vi "Module_UI_SnakeClient.vi"(8 "error in (no error)":errorcluster, 10 "Wait on Module(s) (\"\": none)":string) -> (0 "error out":errorcluster)   [LabVIEW 2019, in "Module_UI_SnakeClient.lvclass"]
doc: "created using\nJSMA Module Template - UI Class 0.3.0.13\nRob Humfeld - Jet Engineering\nCopyright (c) 2020, Jet Engineering"
uses:
  Module_UI_SnakeClient.lvclass
  Private/Module_UI_SnakeClient_jMsgRxList STYP.ctl
  <userlib>/JET Engineering/JSMA Standard Messages/jMsg_Sys_UIPanelOpen/jMsg_Sys_UIPanel_Open.lvclass
  C:/Program Files/National Instruments/LabVIEW 2019/user.lib/Jet Engineering/JSMA/Libraries/jMsg Class/jMsg.lvclass
  Private/Module_UI_SnakeClient_jMsgTxList STYP.ctl
  <userlib>/Jet Engineering/JSMA/Libraries/jMsg_CORE/jMsg_JSMA_ApplicationShutdown/jMsg_JSMA_ApplicationShutdown.lvclass
  C:/Program Files/National Instruments/LabVIEW 2019/user.lib/Jet Engineering/JSMA/Libraries/jModule Class/jModule.lvclass
  Private/Module_UI_SnakeClient_LocalData STYP.ctl
  <userlib>/Jet Engineering/JSMA/Libraries/jModule Class/jModule.lvclass/jModule.ctl
  Module_UI_SnakeClient.lvclass/Module_UI_SnakeClient.ctl
  <userlib>/JET Engineering/JSMA Standard Messages/jMsg_Sys_UIPanelOpen/jMsg_Sys_UIPanel_Open.lvclass/jMsg_Sys_UIPanel_Open.ctl
  <userlib>/Jet Engineering/JET_QSM/Code/Private/JET_QSM - Add State [String API].vi
  <userlib>/Jet Engineering/JET_QSM/Code/Private/JET_QSM - Add State to Front [String API].vi
  <userlib>/Jet Engineering/JSMA/Libraries/jModule Class/jModule - Set Static Timer.vi
  <userlib>/Jet Engineering/JSMA/Libraries/jModule Class/jModule - Set Periodic Timer.vi
  <userlib>/Jet Engineering/JSMA/Libraries/jModule Class/Read jMsgRx.vi
  <vilib>/Utility/error.llb/Trim Whitespace.vi
  <vilib>/Utility/error.llb/Error Cluster From Error Code.vi
  <userlib>/Jet Labs/JET Panel/JETPanel.lvclass
  <userlib>/Jet Engineering/JSMA/Libraries/jModule Class/jModule.lvclass
panel:
  out "winSizer B":string="W"
  out "winSizer A":string="W"
  out "jModule Name":string
  out "Recent states before Error (with tick counts) 2":string="0.167 sec ago: VI Initialize\n0.167 sec ago: Window Open\n0.110 sec ago: Control Update\n0.110 sec ago: Indicator Update\n0.000 sec ago: Error Handler\r\n"
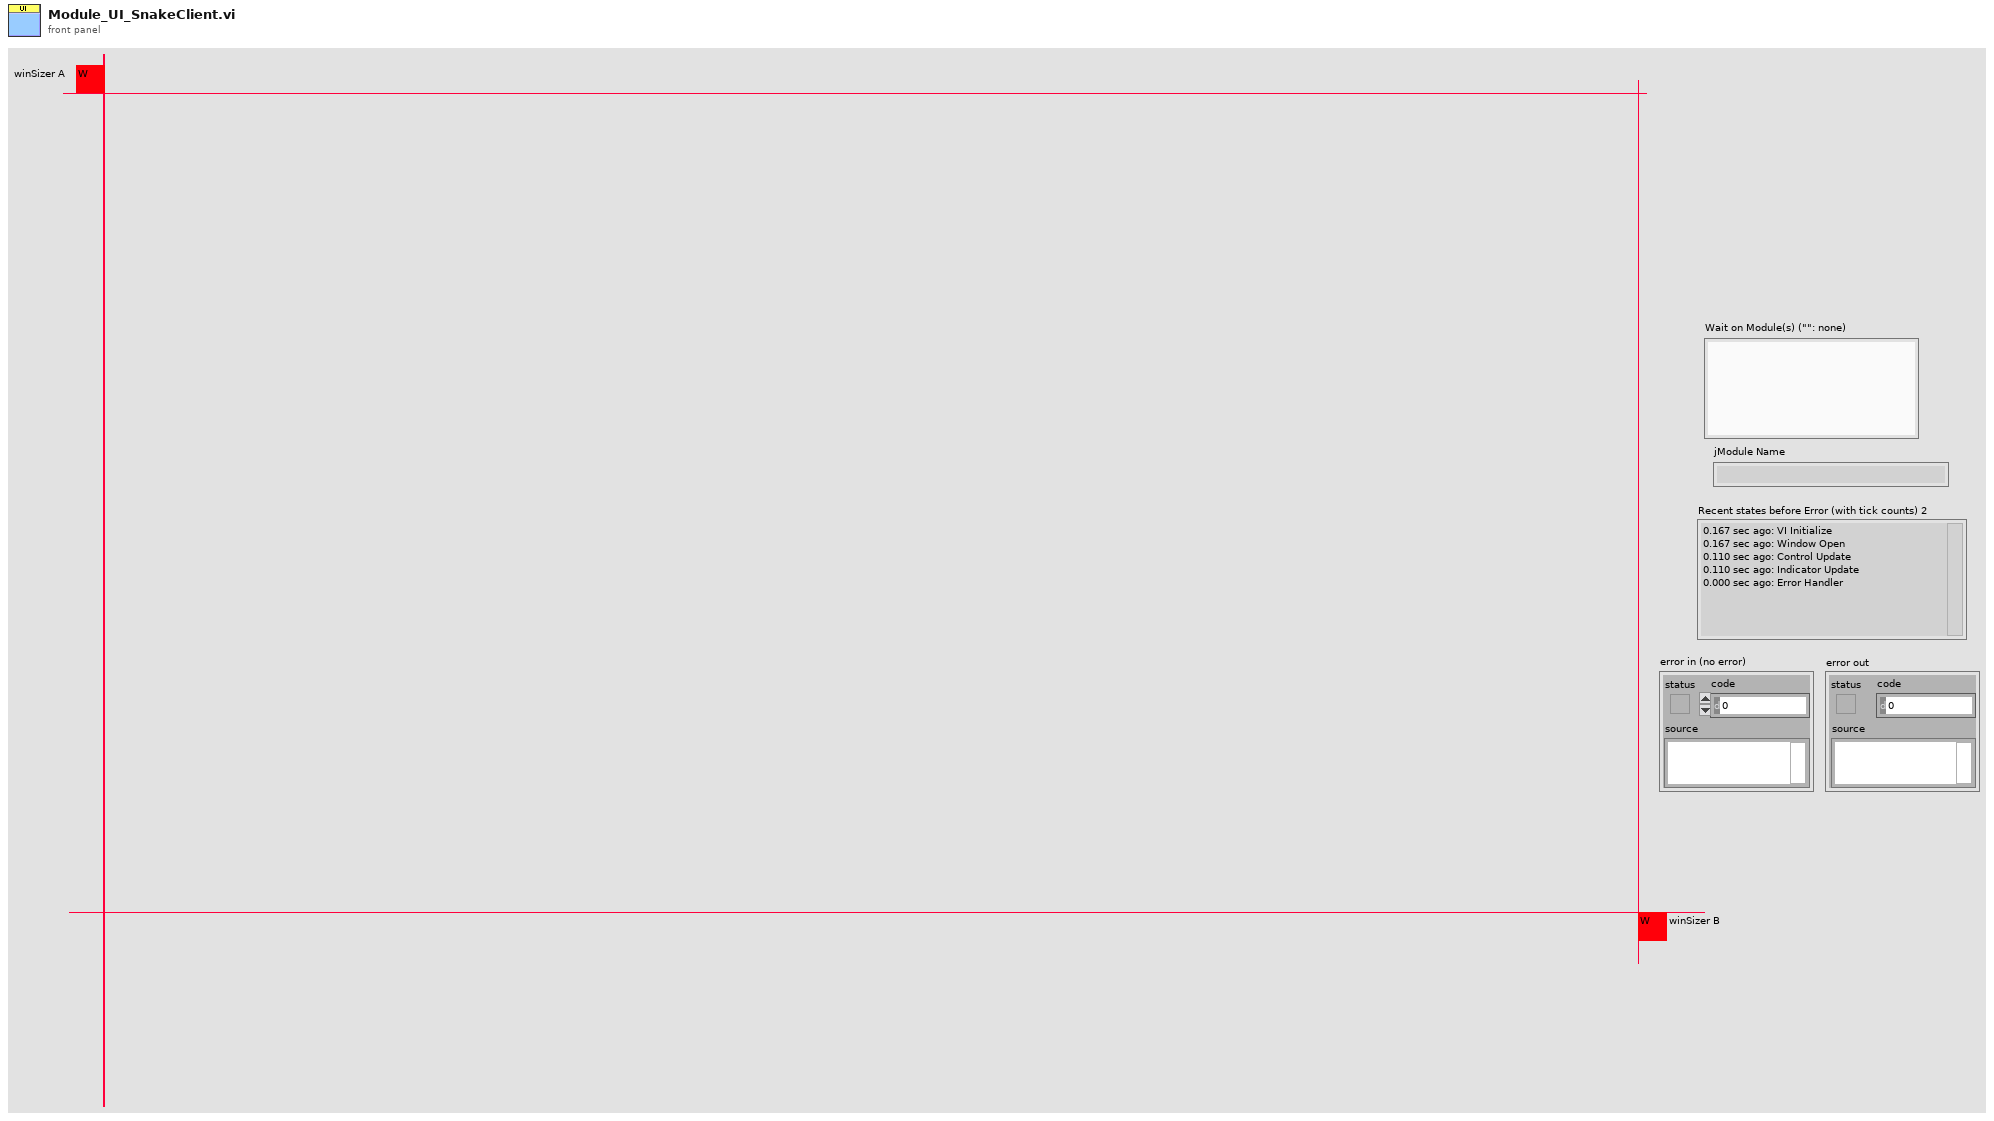
[diagram p1: front panel]
types:
  T1 = typedef "Module_UI_SnakeClient.lvclass/Module_UI_SnakeClient_LocalData STYP.ctl" = cluster{"VI":cluster{"error":errorcluster, "isExiting?":bool}, "UI":cluster{"<placeholder>":bool}}
  T2 = typedef "Module_UI_SnakeClient.lvclass/Module_UI_SnakeClient_jMsgTxList STYP.ctl" = cluster{"jMsg_JSMA_ApplicationShutdown":refnum<class "jMsg_JSMA_ApplicationShutdown.lvclass">}
  T3 = typedef "Module_UI_SnakeClient.lvclass/Module_UI_SnakeClient_jMsgRxList STYP.ctl" = cluster{"jMsg_Sys_UIPanel_Open":refnum<class "jMsg_Sys_UIPanel_Open.lvclass">}
  T4 = typedef "JET_QSM_Refnum STYP.ctl" = cluster{"state":cluster{"queue":refnum<queue>, "idle":string, "error":string, "STOP":string}, "debug":cluster{"enabled?":bool, "queue":refnum<queue>}, "Invalid.option":T5, "QSM.Name":string}
  T5 = typedef "JET_QSM_InvalidOption STYP.ctl" = enum16{"Ignore", "Dialog", "Error"}
  T6 = typedef "JET_QSM_Element STYP.ctl" = cluster{"state":string, "data":variant, "comment":string}
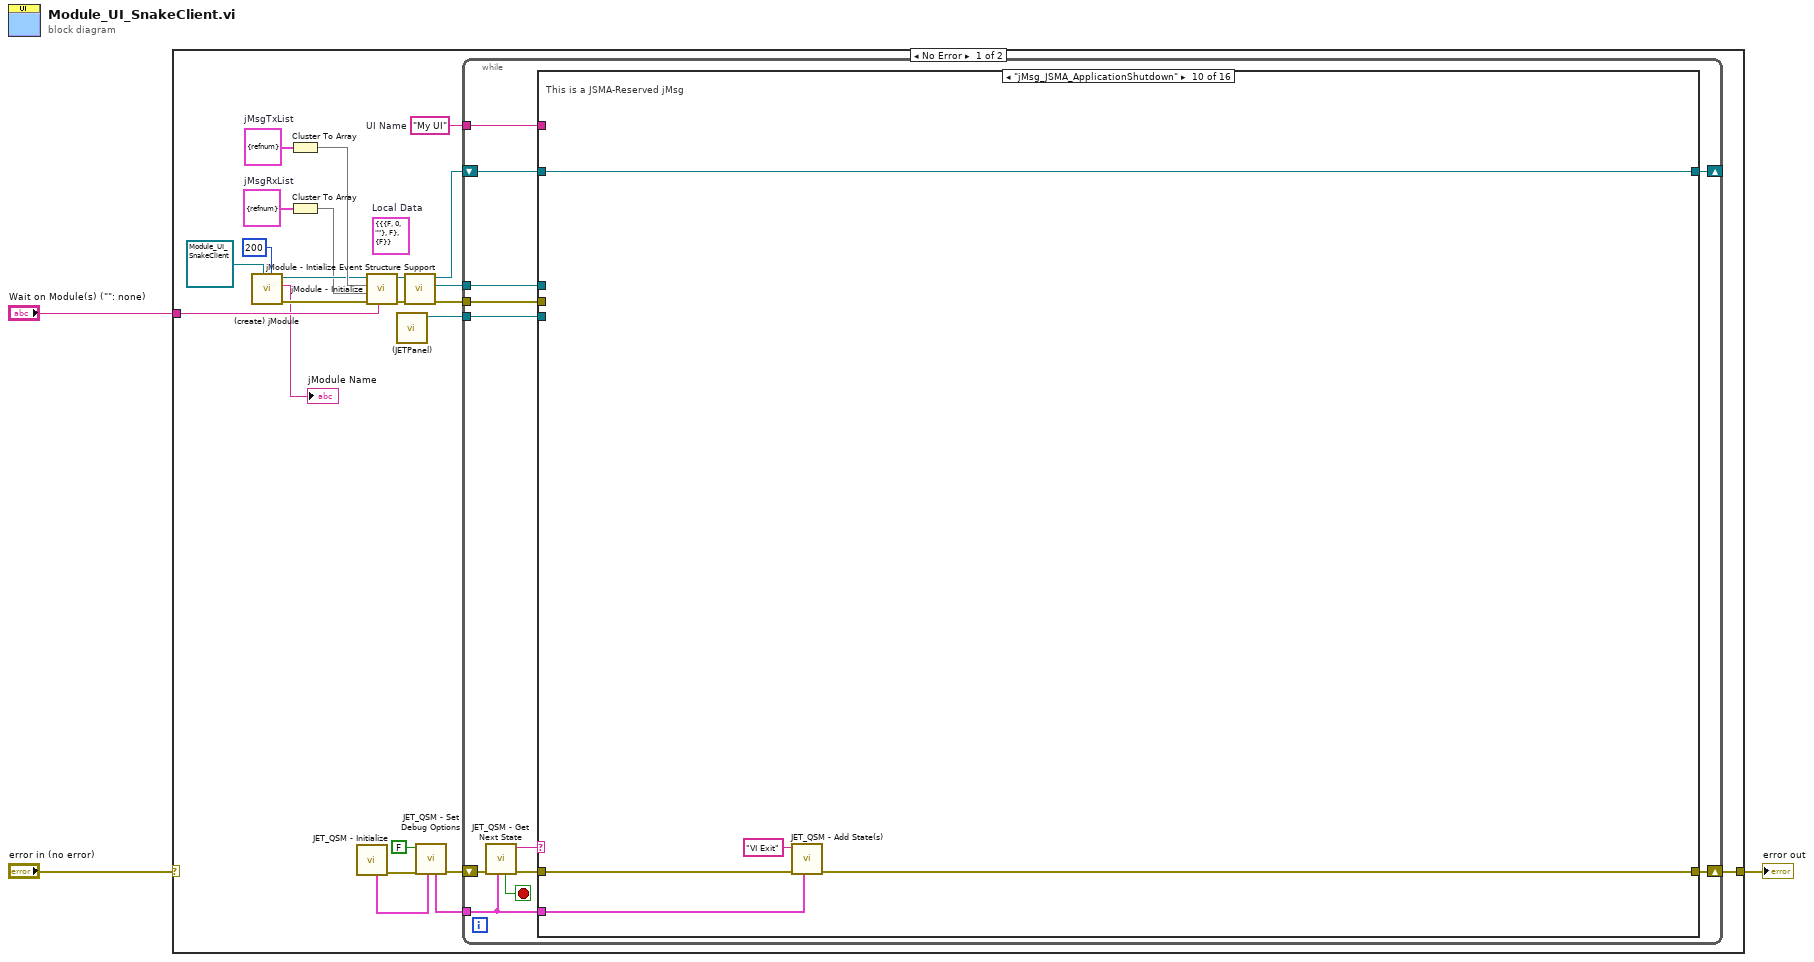
[diagram p0: block diagram]
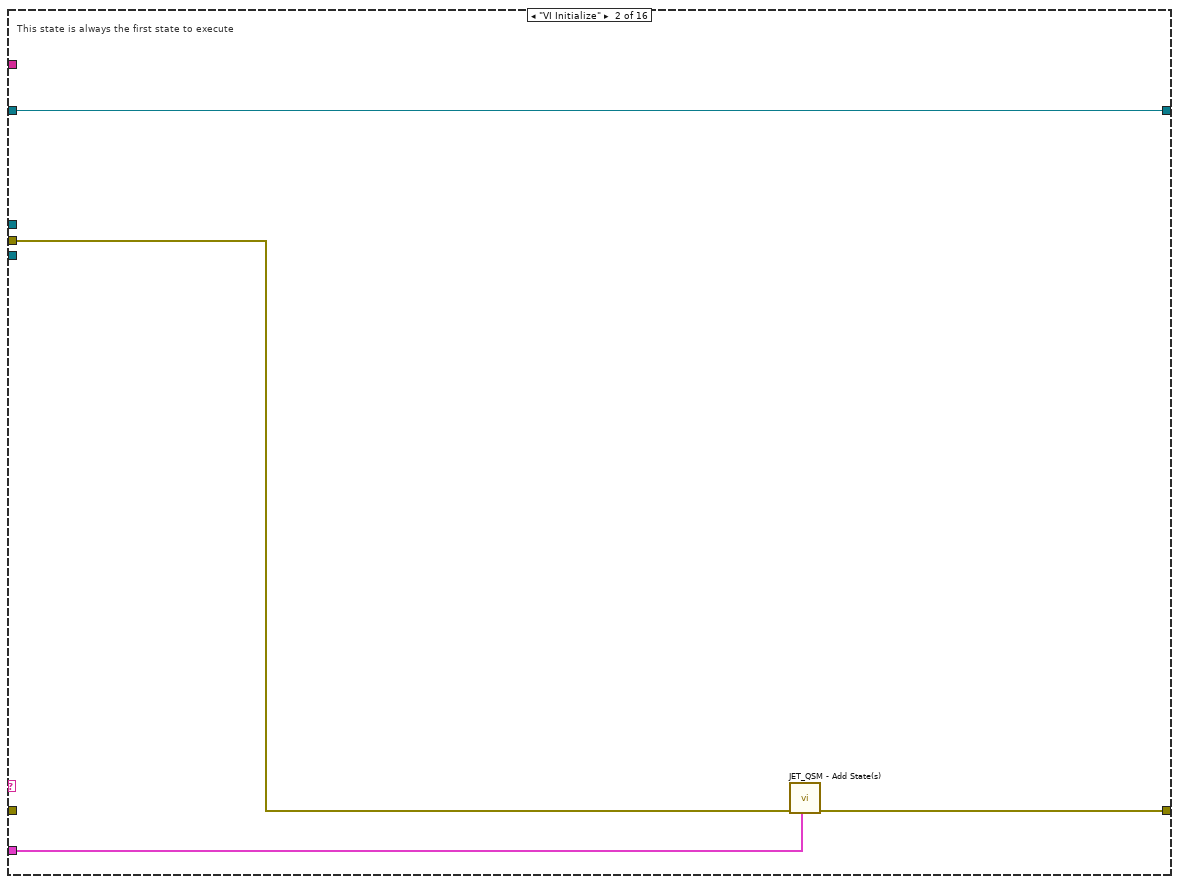
[diagram p3: hidden frame]
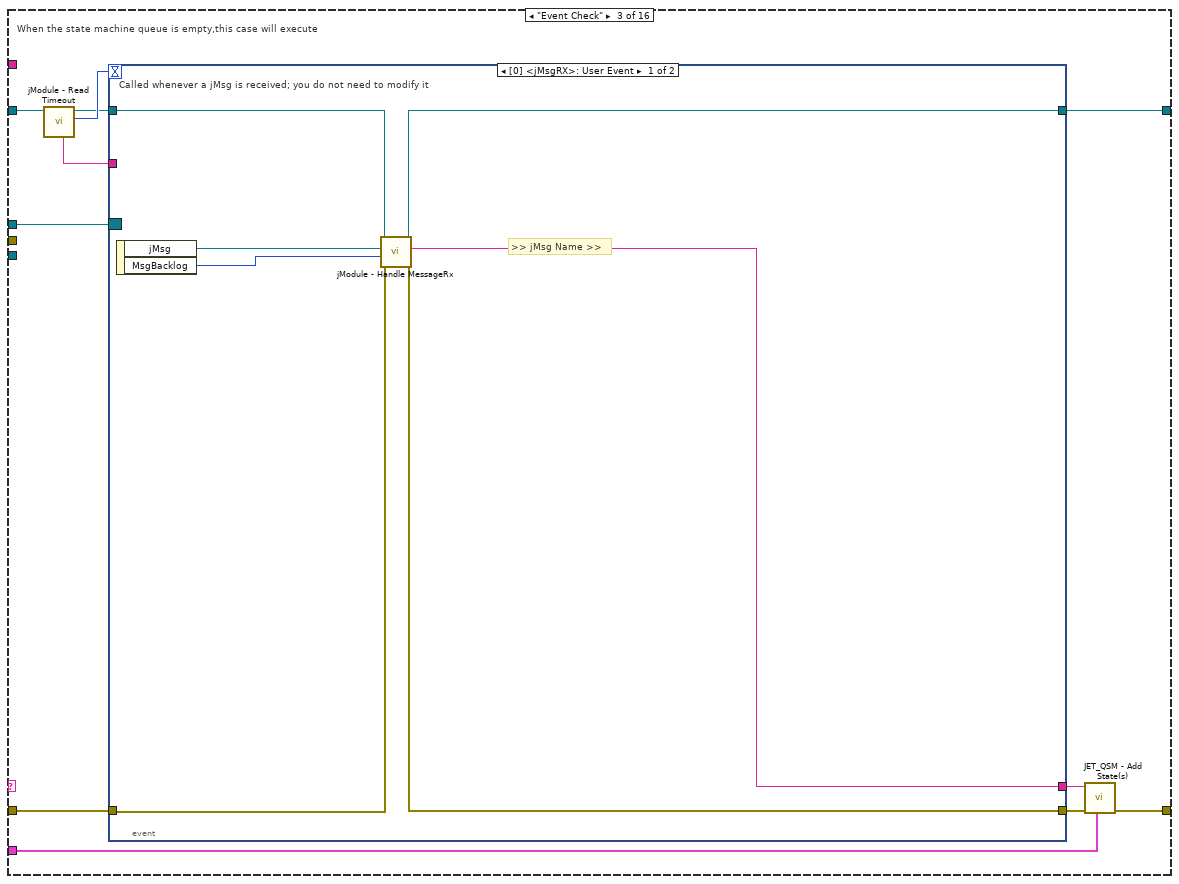
[diagram p4: hidden frame]
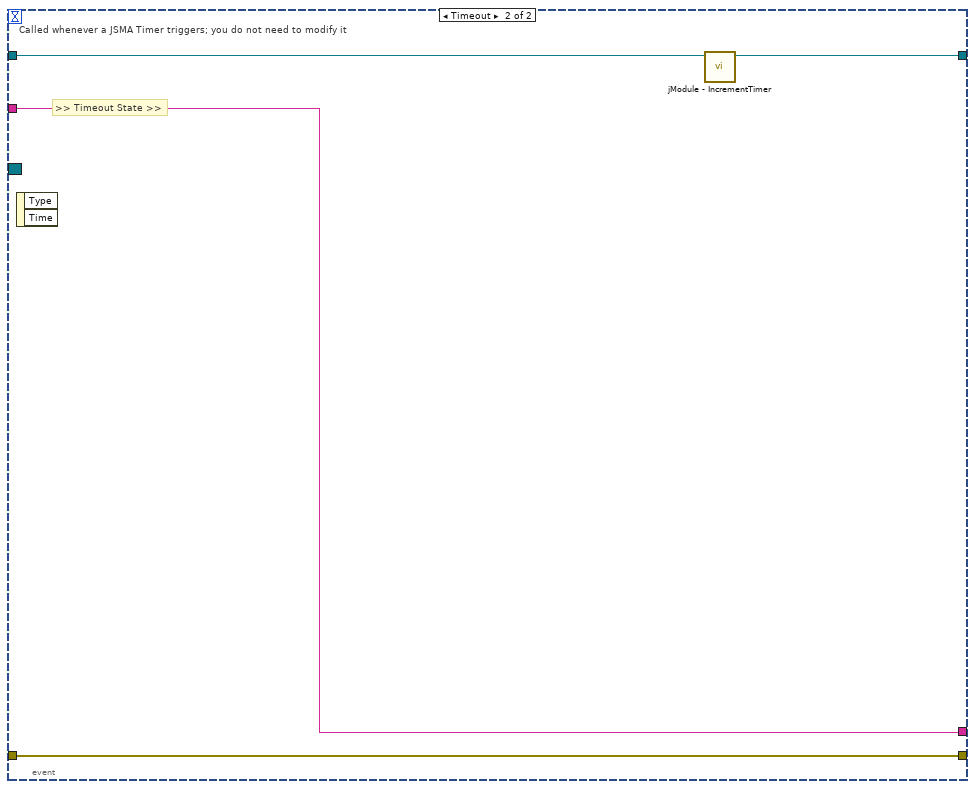
[diagram p5: hidden frame]
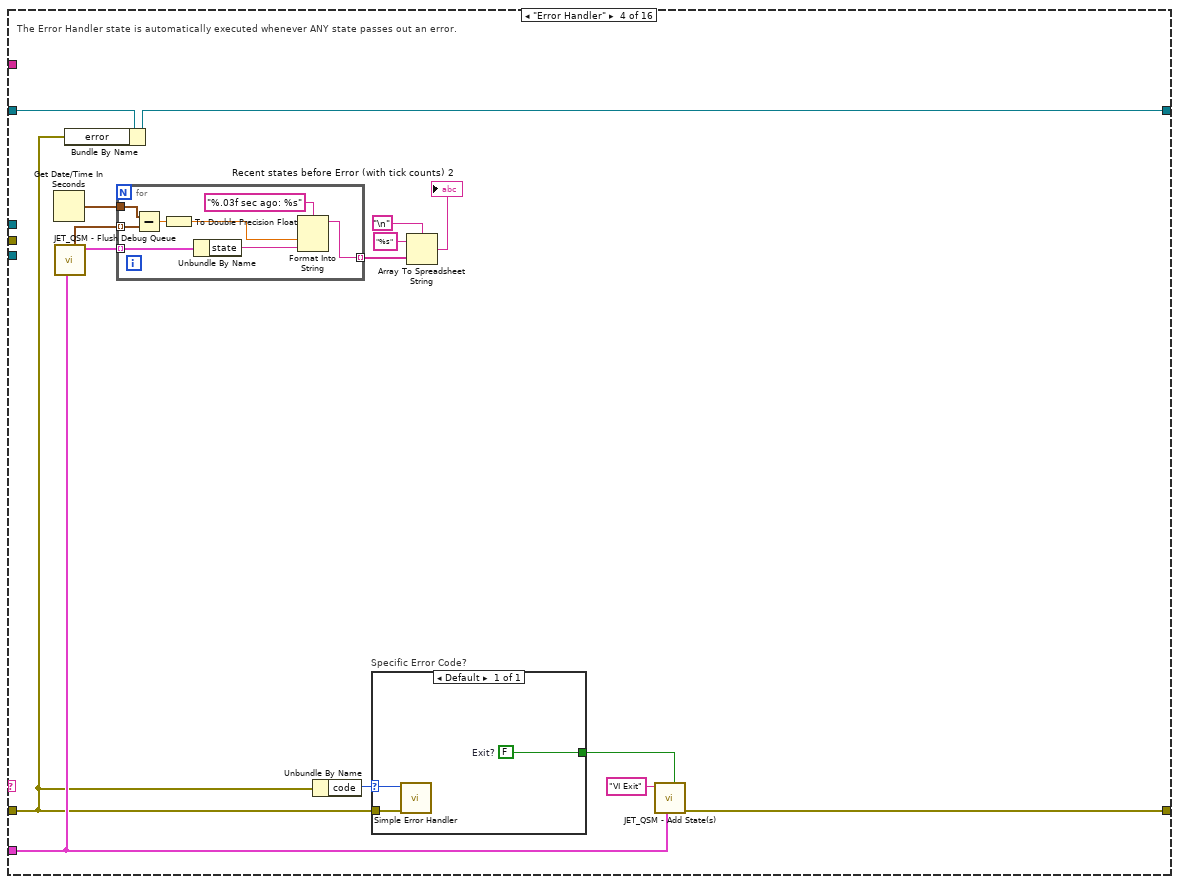
[diagram p6: hidden frame]
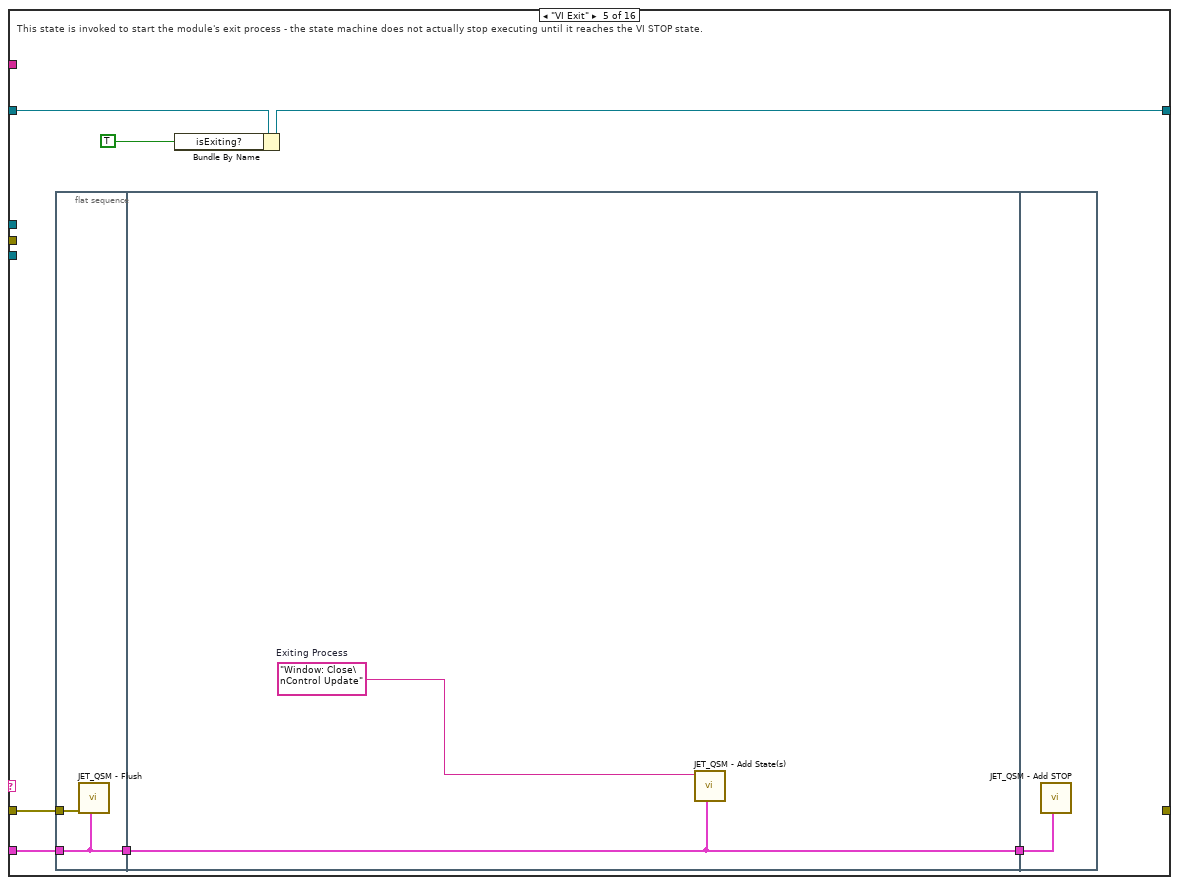
[diagram p7: hidden frame]
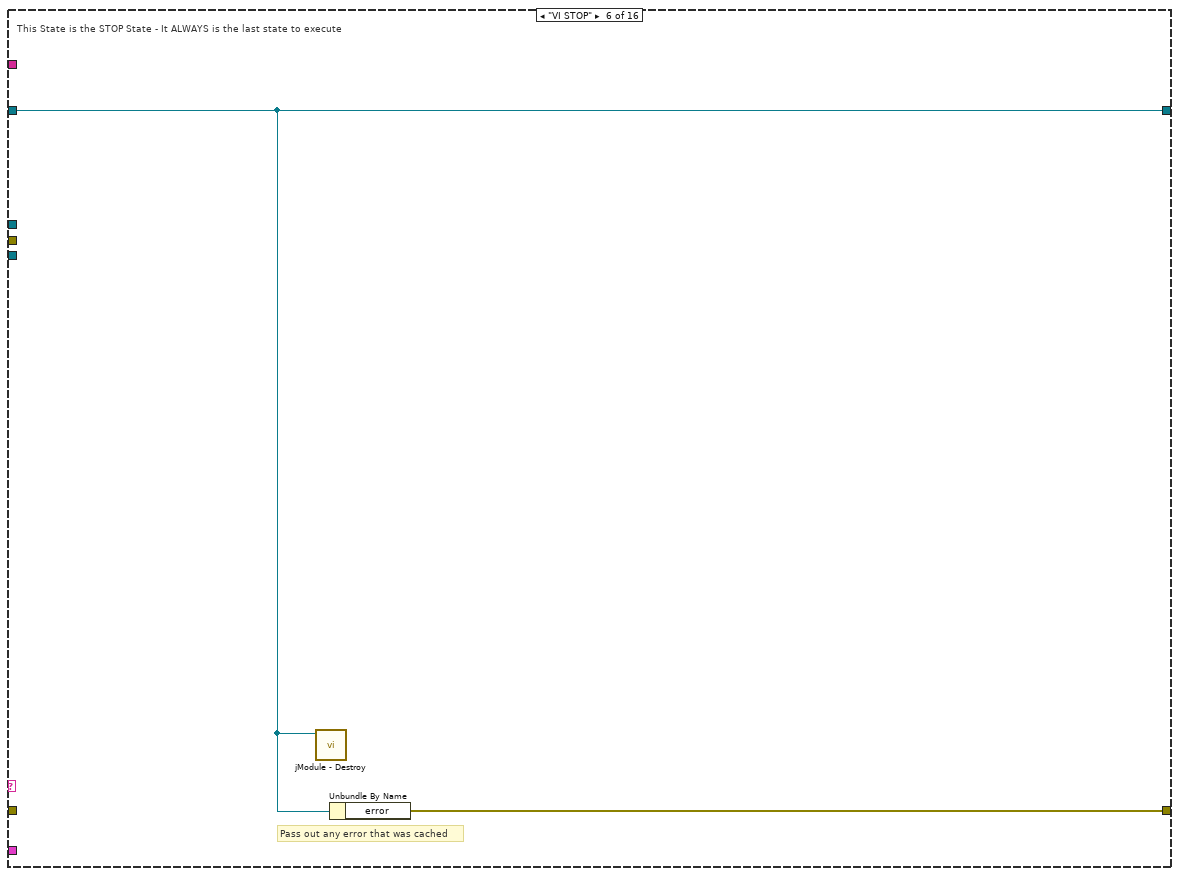
[diagram p8: hidden frame]
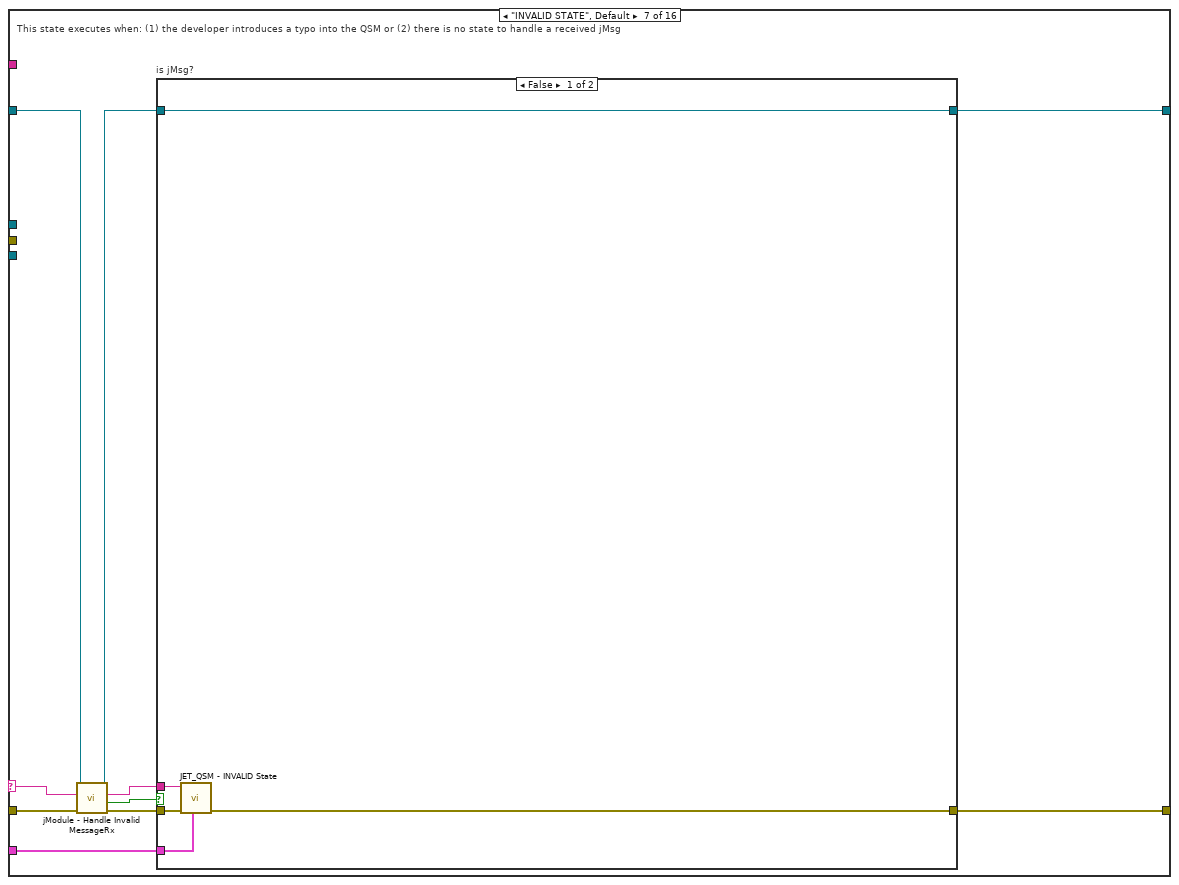
[diagram p9: hidden frame]
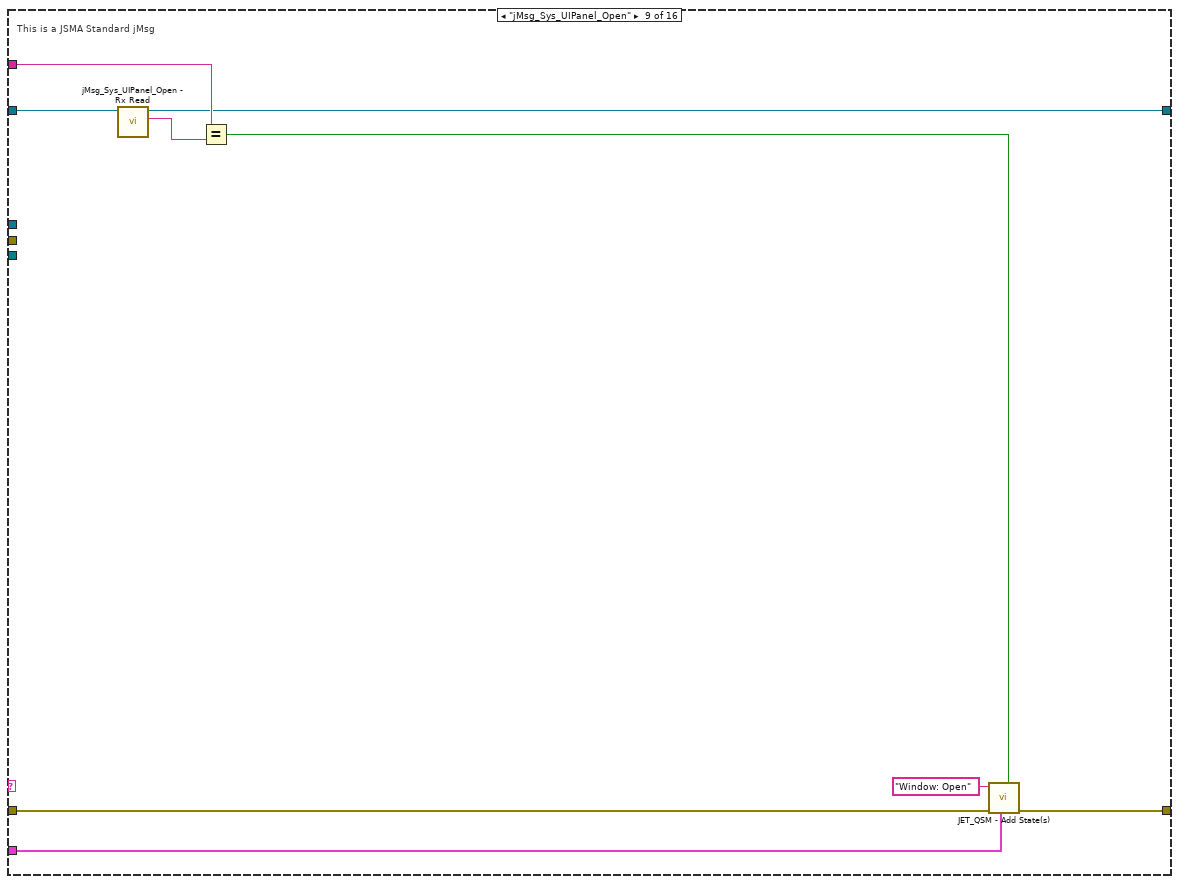
[diagram p12: hidden frame]
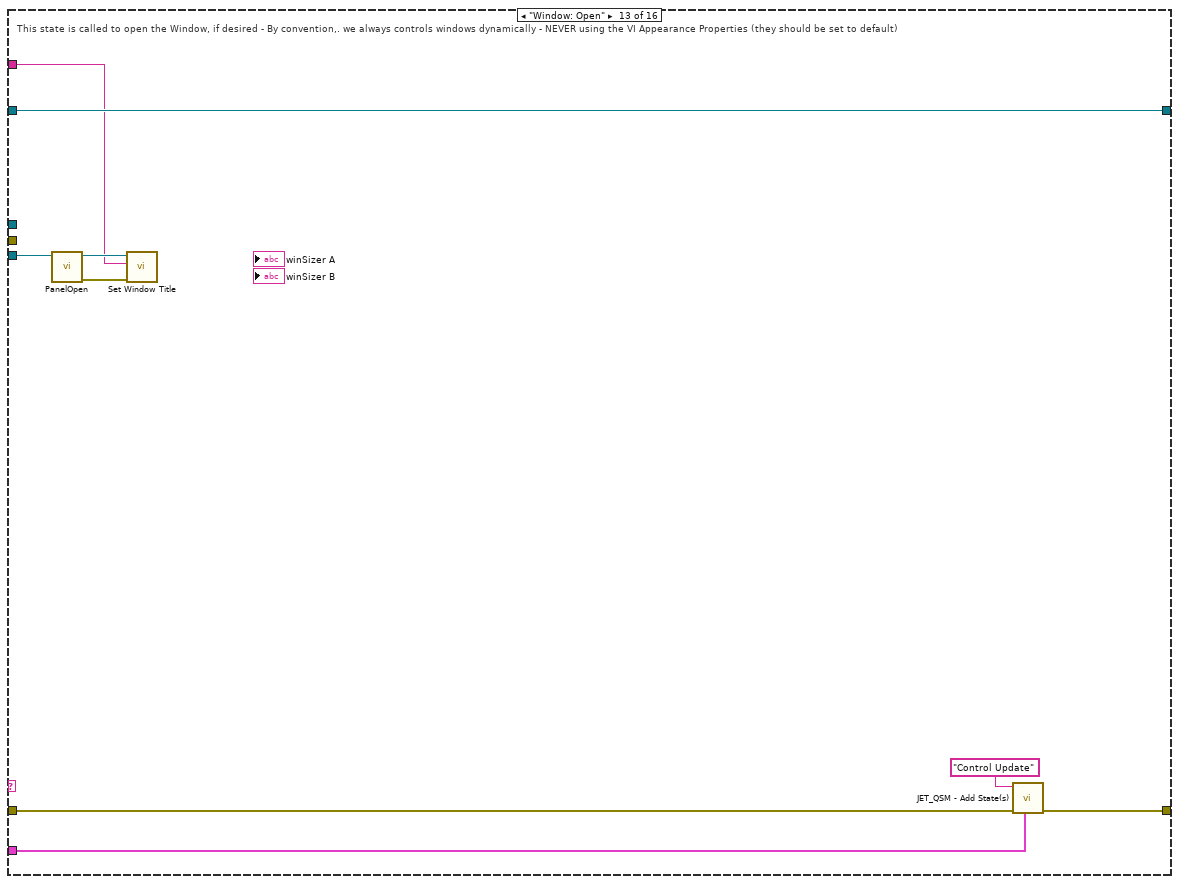
[diagram p15: hidden frame]
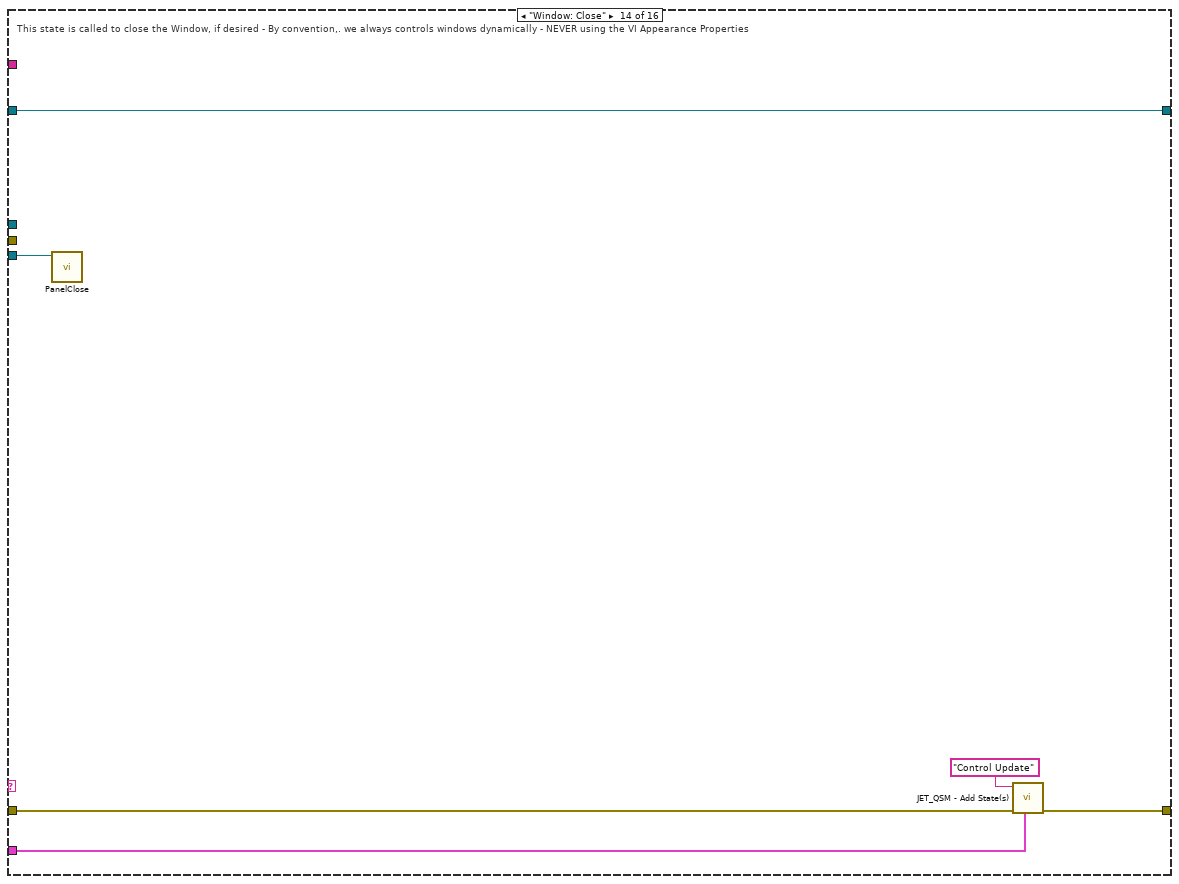
[diagram p16: hidden frame]
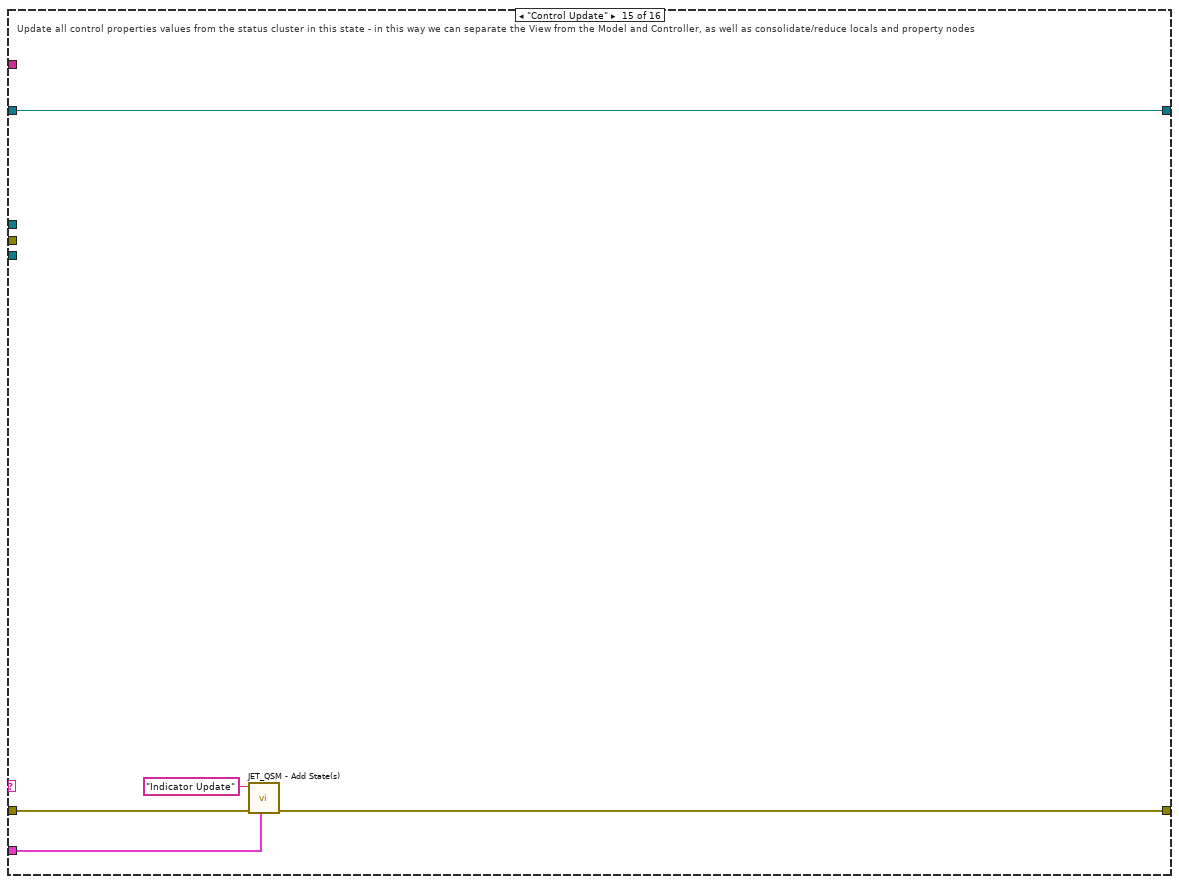
[diagram p17: hidden frame]
diagram:
  n1 = case shown="No Error" "error in (no error)" {
    selector: "error in (no error)" -> [_ w166]
    tunnel: [w26 w166] -> w3
    tunnel: "Wait on Module(s) (\"\": none)" -> [w14 _]
    frame No Error {
      (unwired) T1 {"VI"={"error"={"status"=FALSE, "code"=0, "source"=""}, "isExiting?"=FALSE}, "UI"={"<placeholder>"=FALSE}}  # Local Data
      w13 = T2 {"jMsg_JSMA_ApplicationShutdown"=refnum}  # jMsgTxList
      w12 = T3 {"jMsg_Sys_UIPanel_Open"=refnum}  # jMsgRxList
      w16 = "My UI"  # UI Name
      n2 = call <userlib>:"(create) jModule.vi"("Max Queue size (50)"=200, "jModule Child class"=refnum<class "Module_UI_SnakeClient.lvclass"> refnum ("Module_UI_SystemEventLog.lvclass")) -> ("error out"=w8:errorcluster, "jModule Name"=→"jModule Name":string, "jModule"=w9:refnum<class "Module_UI_SnakeClient.lvclass">)  [unwired: 6 in, 1 out]
      n3 = Cluster To Array(cluster=w13) -> (array=w20:refnum<class "jMsg_JSMA_ApplicationShutdown.lvclass">[])
      n4 = Cluster To Array(cluster=w12) -> (array=w4:refnum<class "jMsg_Sys_UIPanel_Open.lvclass">[])
      n5 = call <userlib>:"JET_QSM - Initialize.vi"() -> ("error out"=w21:errorcluster, "Jet_QSM refnum"=w24:T4)  [unwired: 10 in]
      n6 = call-dynamic "jModule - Initialize.vi"("Wait on Module(s) (\"\": none)"=w14, "error in (no error)"=w8, "jMsgRxList"=w4, "jMsgTxList"=w20, "jModule"=w9) -> ("error out"=w19:errorcluster, "jModule"=w18:refnum<class "Module_UI_SnakeClient.lvclass">)  [unwired: 5 in]
      n7 = call <userlib>:"(JETPanel).vi"() -> ("JETPanel"=w6:refnum<class "JETPanel.lvclass">)  [unwired: 8 in, 3 out]
      n8 = call <userlib>:"jModule - Intialize Event Structure Support.vi"("error in (no error)"=w19, "jModule"=w18) -> ("error out"=w15:errorcluster, "Event Registration Refnum"=w17:refnum<event-registration>, "jModule"=w11:refnum<class "Module_UI_SnakeClient.lvclass">)  [unwired: 6 in, 1 out]
      n9 = call <userlib>:"JET_QSM - Set Debug Options.vi"("Jet_QSM refnum"=w24, "error in (no error)"=w21, "debug.enabled? (F)"=FALSE) -> ("error out"=w22:errorcluster, "Jet_QSM ref"=w23:T4)  [unwired: 7 in]
      n10 = while {
        tunnel: w23 -> [w34]
        shift-right: [w32] -> _
        shift-left: w11 -> [w33]
        shift-right: [w31] -> w26
        shift-left: w22 -> [w38]
        tunnel: w15 -> [w30]
        tunnel: w17 -> [w29]
        tunnel: w16 -> [w28]
        tunnel: w6 -> [w27]
        stop <- w35 stop-if-true
        n11 = call <userlib>:"JET_QSM - Get Next State.vi"("Jet_QSM refnum"=w34, "error in (no error)"=w38) -> ("error out"=w37:errorcluster, "state"=w36:string, "Stop Loop?"=w35:bool)  [unwired: 5 in, 2 out]
        n12 = case shown="\"jMsg_JSMA_ApplicationShutdown\"" w36 {
          selector: w36 -> [_ _ _ _ _ _ w109 _ _ _ _ _ _ _ _ _]
          tunnel: w37 -> [w39 _ w55 w69 w99 _ w111 w124 w131 w135 w140 w142 w148 w154 w162 w165]
          tunnel: w34 -> [_ w44 w54 w73 w98 _ w115 _ w134 w139 _ _ w149 w155 w163 _]
          tunnel: w33 -> [w40 w41 w46 w68 w96 w105 w113 w125 w128 w136 w141 w143 w152 w158 w159 w164]
          tunnel: [w40 w41 w50 w67 w95 w105 w114 w125 w127 w136 w141 w143 w152 w158 w159 w164] -> w32
          tunnel: [w39 w43 w52 w74 _ w106 w116 w124 w133 w138 w140 w142 w147 w153 w161 w165] -> w31
          tunnel: w30 -> [_ w42 _ _ _ _ _ _ _ _ _ _ _ _ _ _]
          tunnel: w29 -> [_ _ w49 _ _ _ _ _ _ _ _ _ _ _ _ _]
          tunnel: w28 -> [_ _ _ _ _ _ _ _ w130 _ _ _ w144 _ _ _]
          tunnel: w27 -> [_ _ _ _ _ _ _ _ _ _ _ _ w151 w157 _ _]
          frame "------ Standard States ------" {
            # "Standard States are required states for a JET_QSM State Machine\n\nTheir names may be changed; see the JET QSM Initialize function to specify the new names"
            # "This is a section header; the state is never expected to execute"
          }
          frame "VI Initialize" {
            # "This state is always the first state to execute"
            n13 = call-poly <userlib>:"JET_QSM - Add State(s).vi"("Jet_QSM refnum"=w44, "error in (no error)"=w42) -> ("error out"=w43:errorcluster)  [unwired: 9 in]
          }
          frame "Event Check" {
            # "When the state machine queue is empty,this case will execute"
            n14 = call <userlib>:"jModule - Read Timeout.vi"("jModule"=w46) -> ("Timeout, ms"=w48:i32, "jModule"=w45:refnum<class "Module_UI_SnakeClient.lvclass">, "Timeout.State"=w47:string)  [unwired: 8 in]
            n15 = event shown="[0] <jMsgRX>: User Event" {
              selector: w49 -> [_ _]
              dyn-events: _ -> [_ _]
              timeout: w48 -> [_ _]
              tunnel: w55 -> [w60 w65]
              tunnel: [w61 w66] -> w53
              tunnel: [w59 w65] -> w51
              tunnel: w45 -> [w57 w64]
              tunnel: [w56 w63] -> w50
              tunnel: w47 -> [_ w66]
              event User Event {
                # ">> jMsg Name >>"
                # "Called whenever a jMsg is received; you do not need to modify it"
                n16 = event-data() -> ("jMsg"=w62:refnum<class "jMsg.lvclass">, "MsgBacklog"=w58:i32)  [unwired: 1 in]
                n17 = call-dynamic "jModule - Handle MessageRx.vi"("error in (no error)"=w60, "Message Backlog"=w58, "jMsg"=w62, "jModule"=w57) -> ("error out"=w59:errorcluster, "QSMState"=w61:string, "jModule"=w56:refnum<class "Module_UI_SnakeClient.lvclass">)  [unwired: 4 in, 1 out]
              }
              event Timeout {
                # ">> Timeout State >>"
                # "Called whenever a JSMA Timer triggers; you do not need to modify it"
                n18 = event-data() -> ()  [unwired: 1 in, 2 out]
                n19 = call <userlib>:"jModule - IncrementTimer.vi"("jModule"=w64) -> ("jModule"=w63:refnum<class "Module_UI_SnakeClient.lvclass">)  [unwired: 10 in]
              }
            }
            n20 = call-poly <userlib>:"JET_QSM - Add State(s).vi"("Jet_QSM refnum"=w54, "error in (no error)"=w51, "state(s)"=w53) -> ("error out"=w52:errorcluster)  [unwired: 8 in]
          }
          frame "Error Handler" {
            # "The Error Handler state is automatically executed whenever ANY state passes out an error."
            n21 = Get Date/Time In Seconds() -> (seconds since 1Jan1904=w77:timestamp)
            n22 = call <userlib>:"JET_QSM - Flush Debug Queue.vi"("Jet_QSM refnum"=w73) -> ("QSM Elements"=w75:T6[], "Timestamps"=w76:timestamp[])  [unwired: 8 in, 1 out]
            n23 = Bundle By Name(cluster=w68, "error"=w69) -> (w67:refnum<class "Module_UI_SnakeClient.lvclass">)
            n24 = for {
              tunnel: w75 -> [w89] mode=indexing
              tunnel: [w87] -> w79 mode=indexing
              tunnel: w77 -> [w84]
              tunnel: w76 -> [w85] mode=indexing
              n25 = Subtract(x=w84, y=w85) -> (x-y=w83:dbl)
              n26 = To Double Precision Float(number=w83) -> (double precision float=w82:dbl)
              n27 = Unbundle By Name(w89) -> ("state"=w88:string)
              n28 = Format Into String(format string="%.03f sec ago: %s", w82, w88) -> (resulting string=w87:string)  [unwired: 2 in, 1 out]
            }
            n29 = Unbundle By Name(w69) -> ("code"=w70:i32)
            n30 = case "Specific Error Code?" shown="Default" w70 {
              selector: w70 -> [w91]
              tunnel: [w92] -> w71
              tunnel: w69 -> [w90]
              frame Default {
                w92 = FALSE  # Exit?
                n31 = call <vilib>:"Simple Error Handler.vi"("error code (no error:0)"=w91, "error in (no error)"=w90) -> ()  [unwired: 3 in, 5 out]
              }
            }
            n32 = Array To Spreadsheet String(delimiter (Tab)="\n", array=w79, 3:"%s" ("format string")) -> (spreadsheet string=→"Recent states before Error (with tick counts) 2":string)
            n33 = call-poly <userlib>:"JET_QSM - Add State(s).vi"("act? (T)"=w71, "Jet_QSM refnum"=w73, "state(s)"="VI Exit") -> ("error out"=w74:errorcluster)  [unwired: 8 in]
          }
          frame "VI Exit" {
            # "This state is invoked to start the module's exit process - the state machine does not actually stop executing until it reaches the VI STOP state."
            n34 = flat-sequence {
              tunnel: w99 -> [w101]
              tunnel: w98 -> [w100]
              tunnel: [w100] -> w97
              tunnel: w97 -> [w103]
              tunnel: [w103] -> w93
              tunnel: w93 -> [w104]
              frame #0 {
                n35 = call <userlib>:"JET_QSM - Flush.vi"("Jet_QSM ref"=w100, "error in (no error)"=w101) -> ()  [unwired: 8 in, 2 out]
              }
              frame #1 {
                w102 = "Window: Close\nControl Update"  # Exiting Process
                n36 = call-poly <userlib>:"JET_QSM - Add State(s).vi"("Jet_QSM refnum"=w103, "state(s)"=w102) -> ()  [unwired: 9 in, 1 out]
              }
              frame #2 {
                n37 = call <userlib>:"JET_QSM - Add STOP.vi"("Jet_QSM refnum"=w104) -> ()  [unwired: 10 in, 1 out]
              }
            }
            n38 = Bundle By Name(cluster=w96, "isExiting?"=TRUE ("VI.isExiting?")) -> (w95:refnum<class "Module_UI_SnakeClient.lvclass">)
          }
          frame "VI STOP" {
            # "Pass out any error that was cached"
            # "This State is the STOP State - It ALWAYS is the last state to execute"
            n39 = call-dynamic "jModule - Destroy.vi"("jModule"=w105) -> ()  [unwired: 10 in, 1 out]
            n40 = Unbundle By Name(w105) -> ("error"=w106:errorcluster)
          }
          frame "INVALID STATE", Default {
            # "This state executes when: (1) the developer introduces a typo into the QSM or (2) there is no state to handle a received jMsg"
            n41 = call-dynamic "jModule - Handle Invalid MessageRx.vi"("error in (no error)"=w111, "Invalid State"=w109, "jModule"=w113) -> ("error out"=w110:errorcluster, "is jMsg State?"=w107:bool, "Invalid State"=w108:string, "jModule"=w112:refnum<class "Module_UI_SnakeClient.lvclass">)  [unwired: 5 in]
            n42 = case "is jMsg?" shown="False" w107 {
              tunnel: [w121 w123] -> w116
              tunnel: w110 -> [w120 w123]
              tunnel: w115 -> [w119 _]
              tunnel: w112 -> [w118 w122]
              tunnel: [w118 w122] -> w114
              tunnel: w108 -> [w117 _]
              frame False {
                n43 = call <userlib>:"JET_QSM - INVALID State.vi"("Jet_QSM refnum"=w119, "error in (no error)"=w120, "state"=w117) -> ("error out"=w121:errorcluster)  [unwired: 8 in]
              }
              frame True {
              }
            }
          }
          frame "------ jMsg  ------" {
            # "This is a section header; the state is never expected to execute"
          }
          frame "jMsg_Sys_UIPanel_Open" {
            # "This is a JSMA Standard jMsg"
            n44 = call <userlib>:"jMsg_Sys_UIPanel_Open - Rx Read.vi"("jModule"=w128) -> ("UI Name"=w126:string, "jModule"=w127:refnum<class "Module_UI_SnakeClient.lvclass">)  [unwired: 6 in, 3 out]
            n45 = Equal?(x=w130, y=w126) -> (x = y?=w129:bool)
            n46 = call-poly <userlib>:"JET_QSM - Add State(s).vi"("act? (T)"=w129, "Jet_QSM refnum"=w134, "error in (no error)"=w131, "state(s)"="Window: Open") -> ("error out"=w133:errorcluster)  [unwired: 7 in]
          }
          frame "jMsg_JSMA_ApplicationShutdown" {
            # "This is a JSMA-Reserved jMsg"
            n47 = call-poly <userlib>:"JET_QSM - Add State(s).vi"("Jet_QSM refnum"=w139, "error in (no error)"=w135, "state(s)"="VI Exit") -> ("error out"=w138:errorcluster)  [unwired: 8 in]
          }
          frame "------ Actions  ------" {
            # "This is a section header; the state is never expected to execute"
          }
          frame "------ Window and Panel Control ------" {
            # "This is a section header; the state is never expected to execute"
          }
          frame "Window: Open" {
            # "This state is called to open the Window, if desired - By convention,. we always controls windows dynamically - NEVER using the VI Appearance Properties (they should be set to default)"
            n48 = call-dynamic "PanelOpen.vi"("JETPanel in"=w151) -> ("error out"=w146:errorcluster, "JETPanel out"=w145:refnum<class "JETPanel.lvclass">)  [unwired: 9 in]
            n49 = call <userlib>:"Set Window Title.vi"("error in (no error)"=w146, "Window Title"=w144, "JETPanel in"=w145) -> ()  [unwired: 7 in, 2 out]
            n50 = call-poly <userlib>:"JET_QSM - Add State(s).vi"("Jet_QSM refnum"=w149, "error in (no error)"=w148, "state(s)"="Control Update") -> ("error out"=w147:errorcluster)  [unwired: 8 in]
          }
          frame "Window: Close" {
            # "This state is called to close the Window, if desired - By convention,. we always controls windows dynamically - NEVER using the VI Appearance Properties"
            n51 = call-dynamic "PanelClose.vi"("JETPanel"=w157) -> ()  [unwired: 9 in, 2 out]
            n52 = call-poly <userlib>:"JET_QSM - Add State(s).vi"("Jet_QSM refnum"=w155, "error in (no error)"=w154, "state(s)"="Control Update") -> ("error out"=w153:errorcluster)  [unwired: 8 in]
          }
          frame "Control Update" {
            # "Update all control properties values from the status cluster in this state - in this way we can separate the View from the Model and Controller, as well as consolidate/reduce locals and property nodes"
            n53 = call-poly <userlib>:"JET_QSM - Add State(s).vi"("Jet_QSM refnum"=w163, "error in (no error)"=w162, "state(s)"="Indicator Update") -> ("error out"=w161:errorcluster)  [unwired: 8 in]
          }
          frame "Indicator Update" {
            # "Update all indicator properties and values from the status cluster in this state - in this way we can separate the View from the Model and Controller, as well as consolidate/reduce property nodes"
          }
        }
      }
    }
    frame Error {
    }
  }
  "error out" <- w3
